vi "Rad Digital Inputs.vi"(8 "error In":errorcluster, 11 "VISA Refnum in":refnum<visa-resource-name>) -> (0 "error out":errorcluster, 2 "Digital Inputs":bool[](array[boolean]), 3 "VISA Refnum out":refnum<visa-resource-name>)   [LabVIEW 2024, in "RaspberryPiPico.lvlib"]
uses:
  RaspberryPiPico.lvlib
  <instrlib>/HandsOnPi2040/HandsOnPi2040.lvlib
  <instrlib>/HandsOnPi2040/Public/DigIns.ctl
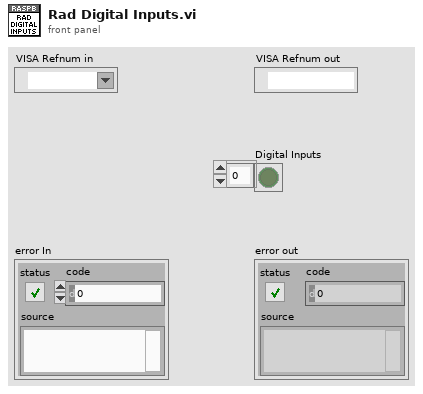
[diagram p1: front panel]
types:
  T1 = typedef "HandsOnPi2040.lvlib/DigIns.ctl" = enum16{"No DI - Error", "DI1 (GPIO7)", "DI2 (GPIO8)", "DI3 (GPIO9)", "DI4 (GPIO10)"}
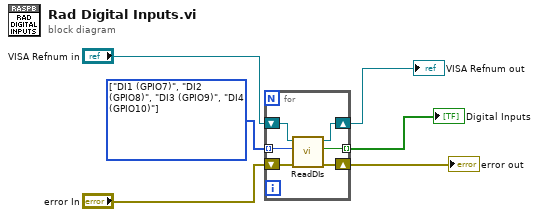
[diagram p0: block diagram]
diagram:
  w2 = T1[] [enum."DI1 (GPIO7)", enum."DI2 (GPIO8)", enum."DI3 (GPIO9)", enum."DI4 (GPIO10)"] items=["No DI - Error", "DI1 (GPIO7)", "DI2 (GPIO8)", "DI3 (GPIO9)", "DI4 (GPIO10)"] ("Array")
  n1 = for {
    shift-right: [w10] -> w4
    shift-left: "VISA Refnum in" -> [w9]
    tunnel: w2 -> [w8] mode=indexing
    shift-right: [w12] -> w5
    shift-left: "error In" -> [w11]
    tunnel: [w7] -> w1 mode=indexing
    n2 = call <instrlib>:"ReadDIs.vi"("error in (no error)"=w11, "Digital Inputs"=w8, "VISA resource name"=w9) -> ("error out"=w12:errorcluster, "DIStatus"=w7:bool, "VISA resource name out"=w10:refnum<visa-resource-name>)  [unwired: 6 in]
  }
  "VISA Refnum out" <- w4
  "error out" <- w5
  "Digital Inputs" <- w1
